vi "test Add Find Remove SLSC Switch CD.vi"(8 "error in (no error)":errorcluster, 11 "TestCase in":refnum<class "SLSC Switch Scripting Unit Tests.lvclass">) -> (0 "error out":errorcluster, 3 "TestCase out":refnum<class "SLSC Switch Scripting Unit Tests.lvclass">)   [LabVIEW 2017, in "SLSC Switch Scripting Unit Tests.lvclass"]
uses:
  SLSC Switch Scripting Unit Tests.lvclass
  SLSC Switch Scripting Unit Tests.lvclass/SLSC Switch Scripting Unit Tests.ctl
  Custom Device/Find All SLSC Switch Custom Devices.vi
  Custom Device/Find SLSC Switch Custom Device by Name.vi
  Custom Device/Find SLSC Switch Custom Device by Slot Number.vi
  <vilib>/addons/_JKI Toolkits/VI Tester/TestCase.llb/TestCase.lvclass
  SLSC Switch Scripting.lvlib
  C:/Program Files (x86)/National Instruments/LabVIEW 2017/vi.lib/addons/_JKI Toolkits/VI Tester/TestCase.llb/TestCase.lvclass
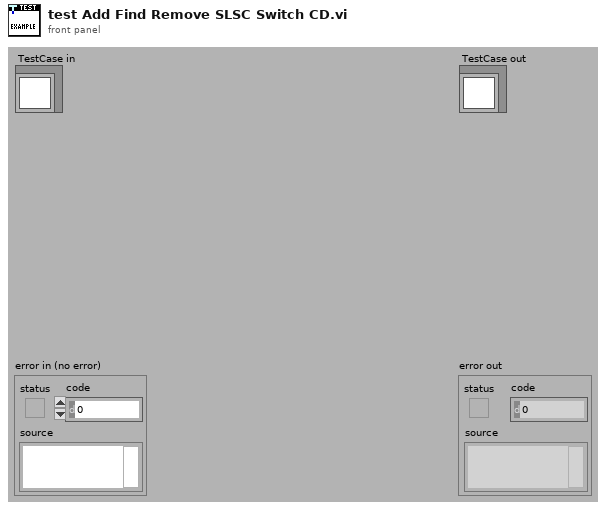
[diagram p1: front panel]
types:
  T1 = typedef "Custom Device API.lvlib/Custom Device Item Ref.ctl" = u64
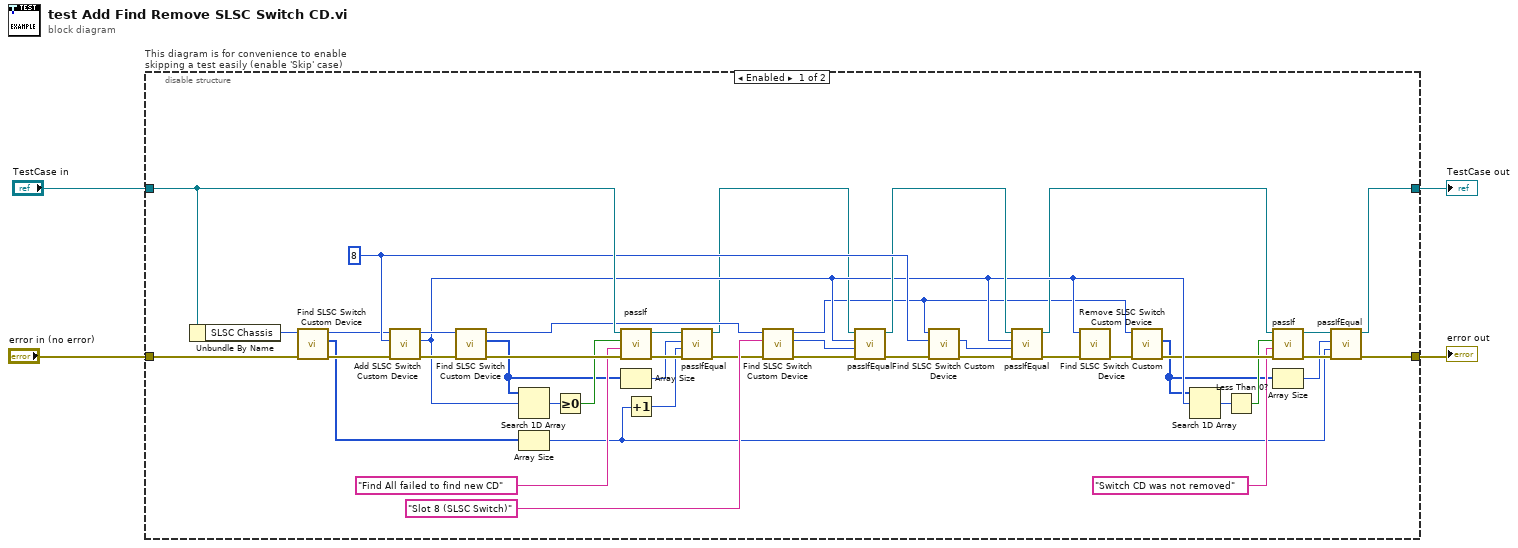
[diagram p0: block diagram]
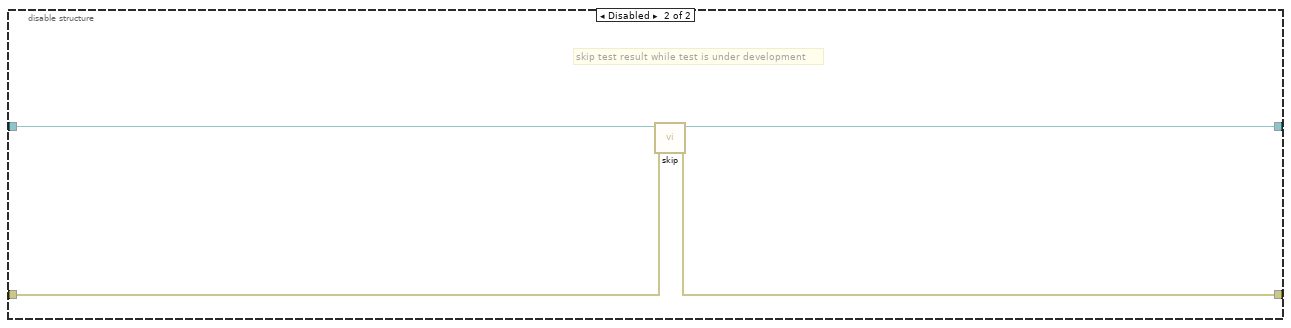
[diagram p2: hidden frame]
diagram:
  n1 = disable-structure "This diagram is for convenience to enable skipping a test easily (enable 'Skip' case)" shown="Enabled" {
    disable-tunnel: "TestCase in" -> [w43 w52]
    disable-tunnel: [w12 w50] -> w1
    disable-tunnel: [w8 w51] -> w3
    disable-tunnel: "error in (no error)" -> [w26 w49]
    frame Enabled {
      w37 = u32 8 ("Slot Number")
      n2 = Unbundle By Name(w43) -> ("SLSC Chassis"=w25:u64)
      n3 = call-poly "Find SLSC Switch Custom Device.vi"("error in (no error)"=w26, "SLSC Chassis Ref"=w25) -> ("error out"=w23:errorcluster, "SLSC Switch Custom Device Ref IDs"=w18:T1[], "SLSC Chassis Ref out"=w24:u64)  [unwired: 7 in]
      n4 = call "Add SLSC Switch Custom Device.vi"("error in (no error)"=w23, "Slot Number"=w37, "SLSC Chassis Ref"=w24) -> ("error out"=w48:errorcluster, "SLSC Switch Custom Device Ref"=w31:T1, "SLSC Chassis Ref out"=w47:u64)  [unwired: 6 in]
      n5 = call-poly "Find SLSC Switch Custom Device.vi"("error in (no error)"=w48, "SLSC Chassis Ref"=w47) -> ("error out"=w46:errorcluster, "SLSC Switch Custom Device Ref IDs"=w16:T1[], "SLSC Chassis Ref out"=w41:u64)  [unwired: 7 in]
      n6 = Search 1D Array(1D array=w16, element=w31) -> (index of element=w45:i32)  [unwired: 1 in]
      n7 = Array Size(array=w18) -> (size(s)=w9:i32)
      n8 = Greater Or Equal To 0?(x=w45) -> (x >= 0?=w44:bool)
      n9 = call-dynamic "passIf.vi"("error in (no error)"=w46, "message (\"\")"="Find All failed to find new CD" ("message (\"\")"), "pass"=w44, "TestCase in"=w43) -> ("error out"=w22:errorcluster, "TestCase out"=w19:refnum<class "SLSC Switch Scripting Unit Tests.lvclass">)  [unwired: 6 in]
      n10 = Array Size(array=w16) -> (size(s)=w17:i32)
      n11 = Increment(x=w9) -> (x+1=w15:i32)
      n12 = call-dynamic "passIfEqual.vi"("error in (no error)"=w22, "y"=w15, "x"=w17, "TestCase in"=w19) -> ("error out"=w21:errorcluster, "TestCase out"=w20:refnum<class "SLSC Switch Scripting Unit Tests.lvclass">)  [unwired: 6 in]
      n13 = call-poly "Find SLSC Switch Custom Device.vi"("error in (no error)"=w21, "Name"="Slot 8 (SLSC Switch)", "SLSC Chassis Ref"=w41) -> ("error out"=w39:errorcluster, "SLSC Switch Custom Device Ref"=w7:T1, "SLSC Chassis Ref out"=w5:u64)  [unwired: 6 in]
      n14 = call-dynamic "passIfEqual.vi"("error in (no error)"=w39, "y"=w7, "x"=w31, "TestCase in"=w20) -> ("error out"=w38:errorcluster, "TestCase out"=w35:refnum<class "SLSC Switch Scripting Unit Tests.lvclass">)  [unwired: 6 in]
      n15 = call-poly "Find SLSC Switch Custom Device.vi"("error in (no error)"=w38, "slot number"=w37, "SLSC Chassis Ref"=w5) -> ("error out"=w36:errorcluster, "SLSC Switch Custom Device Ref"=w6:T1)  [unwired: 6 in, 1 out]
      n16 = call-dynamic "passIfEqual.vi"("error in (no error)"=w36, "y"=w6, "x"=w31, "TestCase in"=w35) -> ("error out"=w34:errorcluster, "TestCase out"=w29:refnum<class "SLSC Switch Scripting Unit Tests.lvclass">)  [unwired: 6 in]
      n17 = call "Remove SLSC Switch Custom Device.vi"("error in (no error)"=w34, "SLSC Switch Custom Device Ref in"=w31) -> ("error out"=w33:errorcluster)  [unwired: 9 in]
      n18 = call-poly "Find SLSC Switch Custom Device.vi"("error in (no error)"=w33, "SLSC Chassis Ref"=w5) -> ("error out"=w30:errorcluster, "SLSC Switch Custom Device Ref IDs"=w11:T1[])  [unwired: 7 in, 1 out]
      n19 = Search 1D Array(1D array=w11, element=w31) -> (index of element=w32:i32)  [unwired: 1 in]
      n20 = Less Than 0?(x=w32) -> (x < 0?=w28:bool)
      n21 = call-dynamic "passIf.vi"("error in (no error)"=w30, "message (\"\")"="Switch CD was not removed" ("message (\"\")"), "pass"=w28, "TestCase in"=w29) -> ("error out"=w14:errorcluster, "TestCase out"=w13:refnum<class "SLSC Switch Scripting Unit Tests.lvclass">)  [unwired: 6 in]
      n22 = Array Size(array=w11) -> (size(s)=w10:i32)
      n23 = call-dynamic "passIfEqual.vi"("error in (no error)"=w14, "y"=w9, "x"=w10, "TestCase in"=w13) -> ("error out"=w8:errorcluster, "TestCase out"=w12:refnum<class "SLSC Switch Scripting Unit Tests.lvclass">)  [unwired: 6 in]
    }
    frame Disabled {
      # "skip test result while test is under development"
      n24 = call <vilib>:"skip.vi"("error in (no error)"=w49, "TestCase in"=w52) -> ("error out"=w51:errorcluster, "TestCase out"=w50:refnum<class "SLSC Switch Scripting Unit Tests.lvclass">)  [unwired: 8 in]
    }
  }
  "error out" <- w3
  "TestCase out" <- w1
